vi "Configure Setpoints Parameters.vi"(7 "Unit Address (1)":u8=1, 8 "error in (no error)":errorcluster, 9 "Setpoint Trim Value (0)":i16, 10 "Setpoint Rate Limit Value (0)":u16, 11 "VISA resource name":refnum<visa-resource-name>) -> (0 "error out":errorcluster, 3 "VISA resource name out":refnum<visa-resource-name>)   [LabVIEW 2014, in "Eurotherm 35xx Series.lvlib"]
doc: "This VI configure setpoints parameters."
uses:
  <instrlib>/Eurotherm 35xx Series/Eurotherm 35xx Series.lvlib
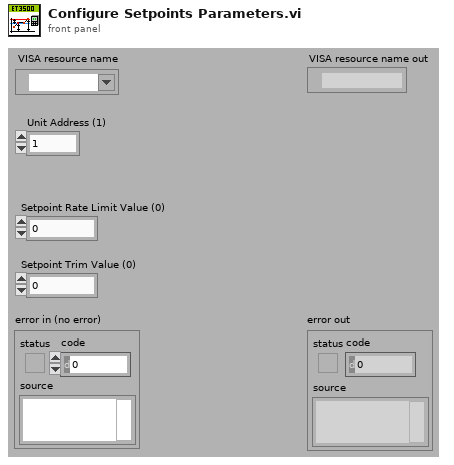
[diagram p1: front panel]
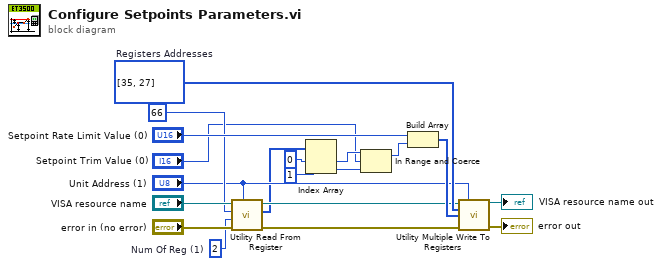
[diagram p0: block diagram]
diagram:
  w11 = u16 2  # Num Of Reg (1)
  w15 = u16[] [35, 27]  # Registers Addresses
  n1 = call <instrlib>:"Utility Read From Register.vi"("Unit Address (1)"="Unit Address (1)", "error in (no error)"="error in (no error)", "Num Of Reg (1)"=w11, "Register Address (0)"=66 ("Register Addresses (0)"), "VISA resource name"="VISA resource name") -> ("error out"=w8:errorcluster, "Data"=w7:i16[], "VISA resource name out"=w9:refnum<visa-resource-name>)  [unwired: 4 in]
  n2 = Index Array(array=w7, index #1=0 ("index"), index #2=1 ("index")) -> (element #1=w4:i16, element #2=w3:i16)
  n3 = In Range and Coerce(upper limit=w4, x="Setpoint Trim Value (0)", lower limit=w3) -> (coerced(x)=w2:i16)  [unwired: 1 out]
  n4 = Build Array("Setpoint Rate Limit Value (0)", w2) -> (w16:u16[])
  n5 = call <instrlib>:"Utility Multiple Write To Registers.vi"("VISA resource name"=w9, "Unit Address (1)"="Unit Address (1)", "Registers Addresses (0)"=w15, "Data (0)"=w16, "error in (no error)"=w8) -> ("VISA resource name out"=→"VISA resource name out":refnum<visa-resource-name>, "error out"=→"error out":errorcluster)  [unwired: 9 in]
